vi "Find Unique Values (Util).vi"(8 "error in (no error)":errorcluster, 11 "Array in":string[](array[string])) -> (0 "error out":errorcluster, 2 "Number repeats for each":i32[](array[numeric]), 3 "Unique Values":string[](array[string]))   [LabVIEW 2019]
doc: "Accepts an array of strings and outputs an array of all unique members and an array of how many occurances each had. \n\n2020 NREL"
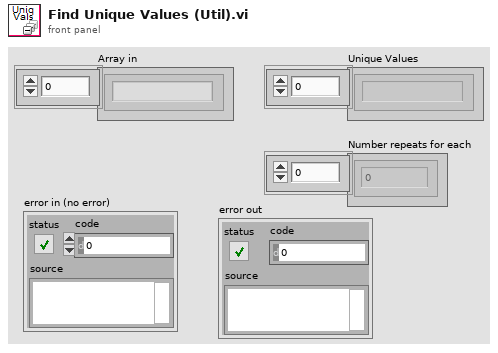
[diagram p1: front panel]
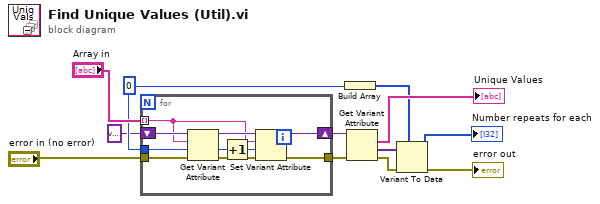
[diagram p0: block diagram]
diagram:
  w9 = 0
  n1 = for {
    tunnel: "Array in" -> [w16] mode=indexing
    shift-right: [w21] -> w8
    shift-left: variant -> [w22]
    tunnel: w9 -> [w17]
    tunnel: [w14] -> w4
    tunnel: "error in (no error)" -> [w13]
    n2 = Get Variant Attribute(Variant=w22, name=w16, default value (empty Variant)=w17, error in=w13) -> (duplicate Variant=w20:variant, value=w19:i32, error out=w15:errorcluster)  [unwired: 1 out]
    n3 = Increment(x=w19) -> (x+1=w18:i32)
    n4 = Set Variant Attribute(Variant=w20, name=w16, value=w18, error in=w15) -> (Variant out=w21:variant, error out=w14:errorcluster)  [unwired: 1 out]
  }
  n5 = Build Array(w9) -> (w7:i32[])
  n6 = Get Variant Attribute(Variant=w8, error in=w4) -> (names=→"Unique Values":string[], values=w6:variant[], error out=w3:errorcluster)  [unwired: 2 in, 1 out]
  n7 = Variant To Data(error in=w3, type=w7, Variant=w6) -> (data=→"Number repeats for each":i32[], error out=→"error out":errorcluster)
